vi "FTW-CSV-Variant-HeaderTraverse.vi"(0 "Variant":variant, 1 "Options":T2={"String Quotes"=FALSE, "Real Format"="%#_15g", "Timestamp Format"="%^<%Y-%m-%dT%H:%M:%S%3uZ>T", "Delimiter"=","}, 5 "Type":T1, 11 "error in":errorcluster) -> (4 "CSV String":string, 15 "error out":errorcluster)   [LabVIEW 2015]
uses:
  FTW-CSV-SerializeOptions.ctl
  <vilib>/Utility/Data Type/Type Definitions/Data Type.ctl
  <vilib>/Utility/Data Type/NI_Data Type.lvlib
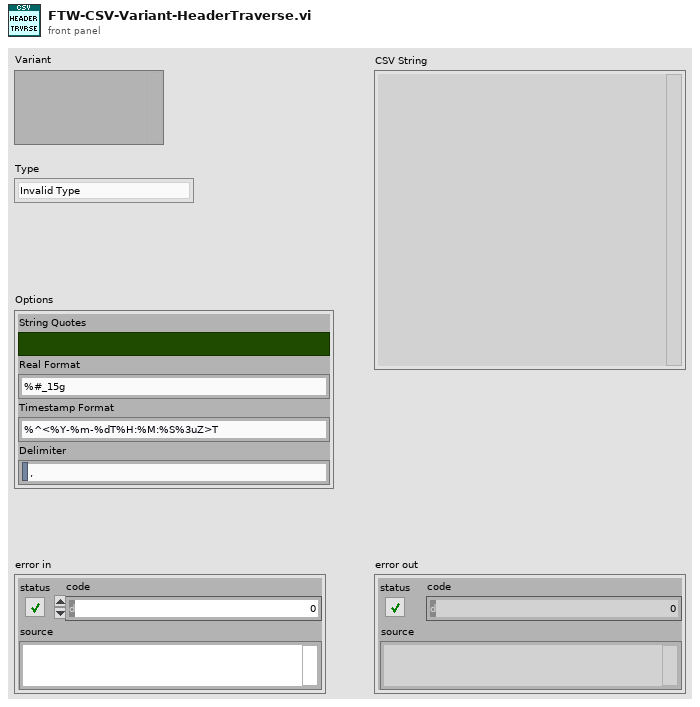
[diagram p1: front panel]
types:
  T1 = typedef "NI_Data Type.lvlib/Data Type.ctl" = enum8{"Invalid Type", "Void", "I8", "I16", "I32", "I64", "U8", "U16", "U32", "U64", "Single Float", "Double Float", "Extended Float", "Single Complex", "Double Complex", "Extended Complex", "Enum U8", "Enum U16", "Enum U32", "Enum U64", "Single Float With Unit", "Double Float With Unit", "Extended Float With Unit", "Single Complex with Unit", "Double Complex with Unit", "Extended Complex with Unit", "Boolean", "String", "Path", "Picture", "Tag", "Array", "Cluster", "Variant", "LV Variant", "Waveform", "Timestamp", "Digital Waveform", "Digital Data", "ExpressData", "Refnum", "External Data", "VI", "Poly VI", "LabVIEW Class Instance", "Fixed Point"}
  T2 = typedef "FTW-CSV-SerializeOptions.ctl" = cluster{"String Quotes":bool, "Real Format":string, "Timestamp Format":string, "Delimiter":string}
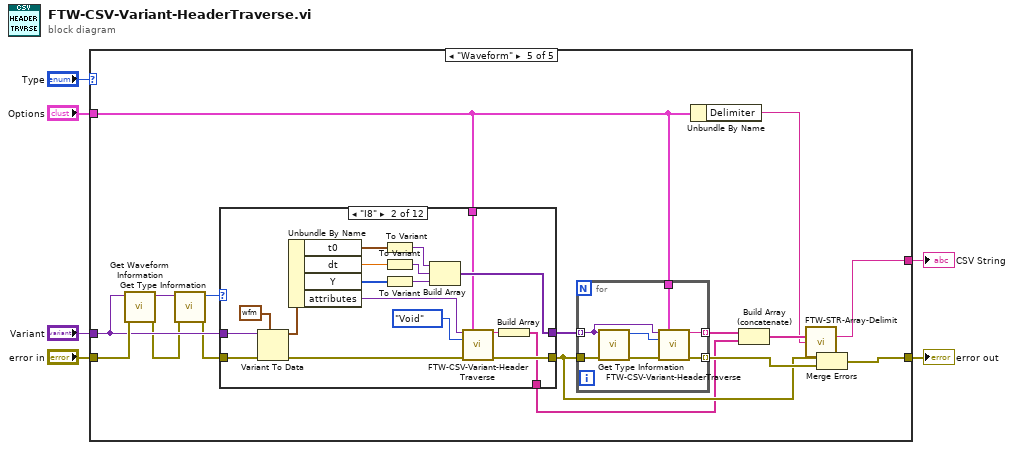
[diagram p0: block diagram]
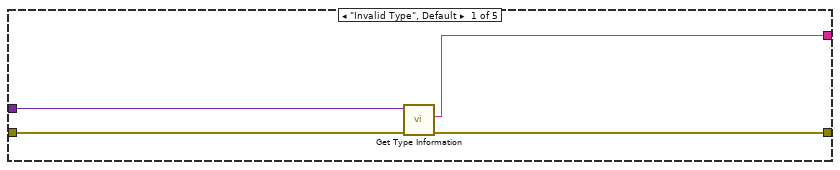
[diagram p2: hidden frame]
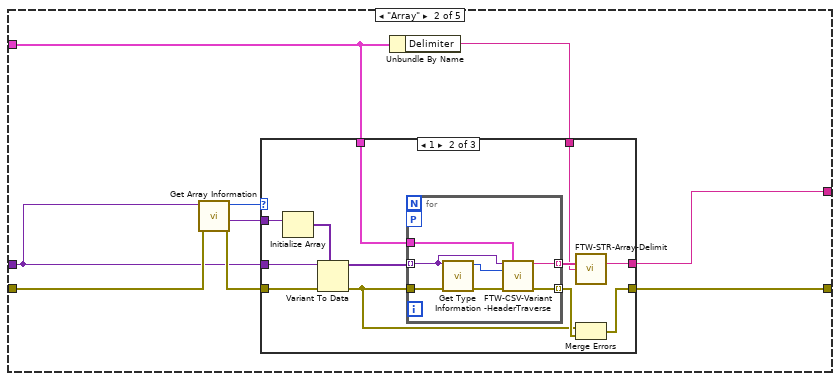
[diagram p3: hidden frame]
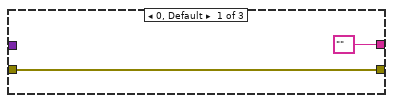
[diagram p4: hidden frame]
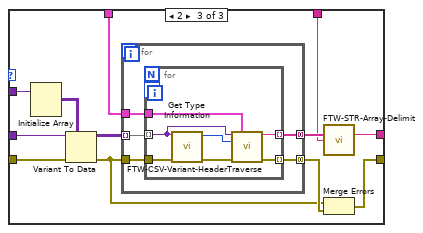
[diagram p5: hidden frame]
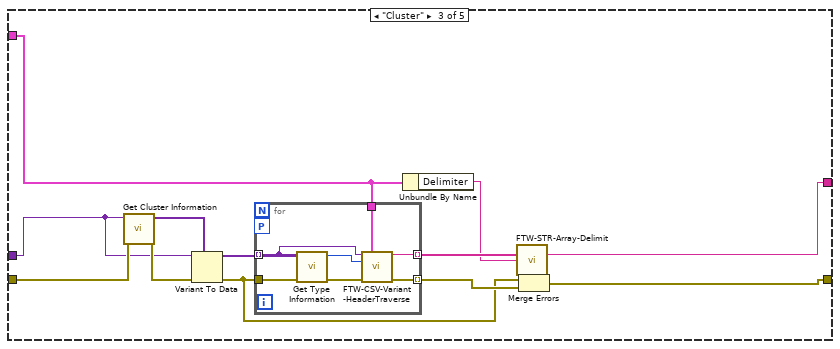
[diagram p6: hidden frame]
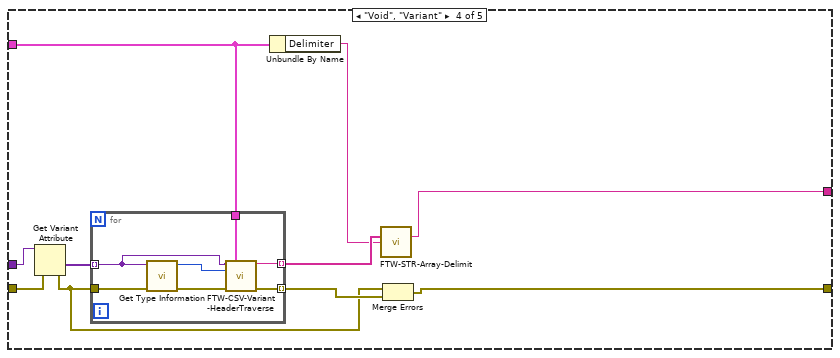
[diagram p7: hidden frame]
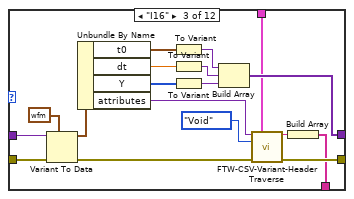
[diagram p9: hidden frame]
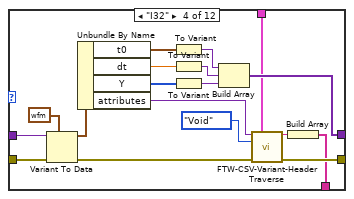
[diagram p10: hidden frame]
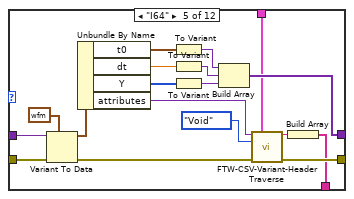
[diagram p11: hidden frame]
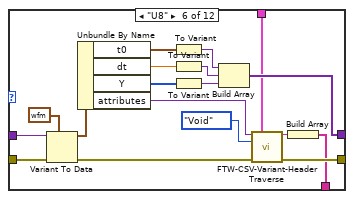
[diagram p12: hidden frame]
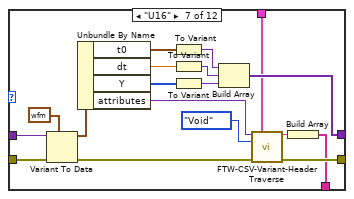
[diagram p13: hidden frame]
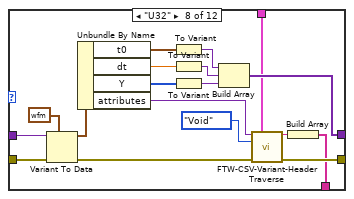
[diagram p14: hidden frame]
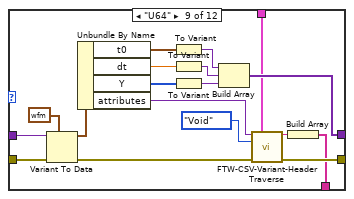
[diagram p15: hidden frame]
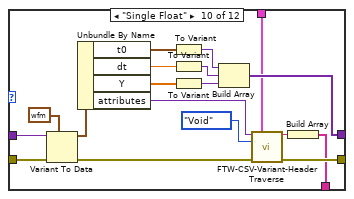
[diagram p16: hidden frame]
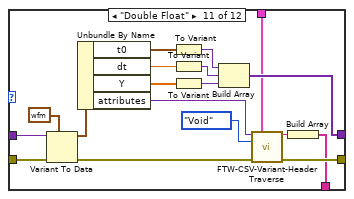
[diagram p17: hidden frame]
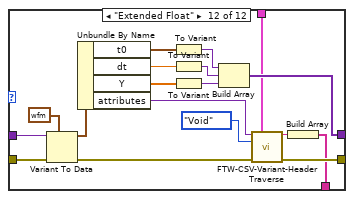
[diagram p18: hidden frame]
diagram:
  n1 = case shown="\"Waveform\"" "Type" {
    tunnel: "error in" -> [w10 w15 w68 w93 w116]
    tunnel: [w9 w14 w65 w89 w112] -> w5
    tunnel: [w7 w13 w66 w90 w113] -> w4
    tunnel: "Variant" -> [w8 w12 w67 w88 w110]
    tunnel: "Options" -> [_ w11 w69 w85 w102]
    frame "Invalid Type", Default {
      n2 = call <vilib>:"Get Type Information.vi"("error in (no error)"=w10, "Variant"=w8) -> ("error out"=w9:errorcluster, "Name"=w7:string)  [unwired: 5 in, 3 out]
    }
    frame "Array" {
      n3 = call <vilib>:"Get Array Information.vi"("error in (no error)"=w15, "Variant"=w12) -> ("error out"=w19:errorcluster, "Array Element Data Type"=w17:variant, "Number of Dimensions"=w18:i32)  [unwired: 6 in, 1 out]
      n4 = Unbundle By Name(w11) -> ("Delimiter"=w16:string)
      n5 = case shown="1" w18 {
        tunnel: [w21 w25 w44] -> w14
        tunnel: w19 -> [w21 w32 w51]
        tunnel: w17 -> [_ w28 w47]
        tunnel: ["" ("empty string") w30 w49] -> w13
        tunnel: w12 -> [_ w29 w48]
        tunnel: w11 -> [_ w23 w42]
        tunnel: w16 -> [_ w22 w41]
        frame 0, Default {
        }
        frame 1 {
          n6 = Initialize Array(w28) -> (w27:variant[])  [unwired: 1 in]
          n7 = Variant To Data(error in=w32, type=w27, Variant=w29) -> (data=w26:variant[], error out=w24:errorcluster)
          n8 = for {
            tunnel: w26 -> [w35] mode=indexing
            tunnel: [w39] -> w31 mode=indexing
            tunnel: w24 -> [w38]
            tunnel: [w40] -> w33 mode=indexing
            tunnel: w23 -> [w37]
            workers-P: _ -> [_]
            n9 = call <vilib>:"Get Type Information.vi"("error in (no error)"=w38, "Variant"=w35) -> ("error out"=w36:errorcluster, "Type"=w34:T1)  [unwired: 5 in, 3 out]
            n10 = call "FTW-CSV-Variant-HeaderTraverse.vi"("Variant"=w35, "Options"=w37, "Type"=w34, "error in"=w36) -> ("CSV String"=w39:string, "error out"=w40:errorcluster)  [unwired: 10 in]
          }
          n11 = call "FTW-STR-Array-Delimit.vi"("Array of Strings"=w31, "Delimiter"=w22) -> ("Delimited String"=w30:string)  [unwired: 13 in]
          n12 = Merge Errors(w24, w33) -> (w25:errorcluster)
        }
        frame 2 {
          n13 = Initialize Array(w47) -> (w46:variant[][])  [unwired: 2 in]
          n14 = Variant To Data(error in=w51, type=w46, Variant=w48) -> (data=w45:variant[][], error out=w43:errorcluster)
          n15 = for {
            tunnel: [w57] -> w52 mode=concatenating
            tunnel: [w56] -> w50 mode=concatenating
            tunnel: w45 -> [w55] mode=indexing
            tunnel: w43 -> [w54]
            tunnel: w42 -> [w53]
            n16 = for {
              tunnel: w55 -> [w59] mode=indexing
              tunnel: [w63] -> w56 mode=indexing
              tunnel: w54 -> [w62]
              tunnel: [w64] -> w57 mode=indexing
              tunnel: w53 -> [w61]
              workers-P: _ -> [_]
              n17 = call <vilib>:"Get Type Information.vi"("error in (no error)"=w62, "Variant"=w59) -> ("error out"=w60:errorcluster, "Type"=w58:T1)  [unwired: 5 in, 3 out]
              n18 = call "FTW-CSV-Variant-HeaderTraverse.vi"("Variant"=w59, "Options"=w61, "Type"=w58, "error in"=w60) -> ("CSV String"=w63:string, "error out"=w64:errorcluster)  [unwired: 10 in]
            }
          }
          n19 = call "FTW-STR-Array-Delimit.vi"("Array of Strings"=w50, "Delimiter"=w41) -> ("Delimited String"=w49:string)  [unwired: 13 in]
          n20 = Merge Errors(w43, w52) -> (w44:errorcluster)
        }
      }
    }
    frame "Cluster" {
      n21 = call <vilib>:"Get Cluster Information.vi"("error in (no error)"=w68, "Variant"=w67) -> ("error out"=w74:errorcluster, "Cluster Elements"=w72:variant[])  [unwired: 8 in]
      n22 = Variant To Data(error in=w74, type=w72, Variant=w67) -> (data=w71:variant[], error out=w73:errorcluster)
      n23 = for {
        tunnel: w71 -> [w78] mode=indexing
        tunnel: [w81] -> w75 mode=indexing
        tunnel: w73 -> [w83]
        tunnel: [w82] -> w76 mode=indexing
        tunnel: w69 -> [w80]
        workers-P: _ -> [_]
        n24 = call <vilib>:"Get Type Information.vi"("error in (no error)"=w83, "Variant"=w78) -> ("error out"=w79:errorcluster, "Type"=w77:T1)  [unwired: 5 in, 3 out]
        n25 = call "FTW-CSV-Variant-HeaderTraverse.vi"("Variant"=w78, "Options"=w80, "Type"=w77, "error in"=w79) -> ("CSV String"=w81:string, "error out"=w82:errorcluster)  [unwired: 10 in]
      }
      n26 = Unbundle By Name(w69) -> ("Delimiter"=w70:string)
      n27 = call "FTW-STR-Array-Delimit.vi"("Array of Strings"=w75, "Delimiter"=w70) -> ("Delimited String"=w66:string)  [unwired: 13 in]
      n28 = Merge Errors(w73, w76) -> (w65:errorcluster)
    }
    frame "Void", "Variant" {
      n29 = Get Variant Attribute(Variant=w88, error in=w93) -> (values=w86:variant[], error out=w87:errorcluster)  [unwired: 2 in, 2 out]
      n30 = for {
        tunnel: w86 -> [w95] mode=indexing
        tunnel: [w99] -> w91 mode=indexing
        tunnel: w87 -> [w97]
        tunnel: [w100] -> w92 mode=indexing
        tunnel: w85 -> [w98]
        n31 = call <vilib>:"Get Type Information.vi"("error in (no error)"=w97, "Variant"=w95) -> ("error out"=w96:errorcluster, "Type"=w94:T1)  [unwired: 5 in, 3 out]
        n32 = call "FTW-CSV-Variant-HeaderTraverse.vi"("Variant"=w95, "Options"=w98, "Type"=w94, "error in"=w96) -> ("CSV String"=w99:string, "error out"=w100:errorcluster)  [unwired: 10 in]
      }
      n33 = Unbundle By Name(w85) -> ("Delimiter"=w84:string)
      n34 = call "FTW-STR-Array-Delimit.vi"("Array of Strings"=w91, "Delimiter"=w84) -> ("Delimited String"=w90:string)  [unwired: 13 in]
      n35 = Merge Errors(w87, w92) -> (w89:errorcluster)
    }
    frame "Waveform" {
      n36 = call <vilib>:"Get Waveform Information.vi"("error in (no error)"=w116, "Variant"=w110) -> ("error out"=w107:errorcluster, "Y Array Type"=w108:variant)  [unwired: 8 in]
      n37 = call <vilib>:"Get Type Information.vi"("error in (no error)"=w107, "Variant"=w108) -> ("error out"=w106:errorcluster, "Type"=w105:T1)  [unwired: 5 in, 3 out]
      n38 = case shown="\"I8\"" w105 {
        tunnel: [w117 w123 w141 w159 w177 w195 w213 w231 w249 w267 w285 w303] -> w111
        tunnel: w110 -> [_ w127 w145 w163 w181 w199 w217 w235 w253 w271 w289 w307]
        tunnel: [_ w135 w153 w171 w189 w207 w225 w243 w261 w279 w297 w315] -> w109
        tunnel: w106 -> [w117 w131 w149 w167 w185 w203 w221 w239 w257 w275 w293 w311]
        tunnel: w102 -> [_ w122 w140 w158 w176 w194 w212 w230 w248 w266 w284 w302]
        tunnel: [_ w118 w136 w154 w172 w190 w208 w226 w244 w262 w280 w298] -> w103
        frame "Invalid Type", Default {
        }
        frame "I8" {
          n39 = Variant To Data(error in=w131, type=waveform(i8) {"t0"=timestamp(0 s since 1904-01-01), "dt"=1.0, "Y"=[]} ("Waveform"), Variant=w127) -> (data=w125:waveform(i8), error out=w124:errorcluster)
          n40 = Unbundle By Name(w125) -> ("t0"=w130:timestamp, "dt"=w129:dbl, "Y"=w128:i8[], "attributes"=w121:variant)
          n41 = To Variant(anything=w130) -> (Variant=w134:variant)
          n42 = To Variant(anything=w129) -> (Variant=w133:variant)
          n43 = To Variant(anything=w128) -> (Variant=w132:variant)
          n44 = Build Array(w134, w133, w132) -> (w135:variant[])
          n45 = call "FTW-CSV-Variant-HeaderTraverse.vi"("Variant"=w121, "Options"=w122, "Type"=Data_Type."Void", "error in"=w124) -> ("CSV String"=w119:string, "error out"=w123:errorcluster)  [unwired: 10 in]
          n46 = Build Array(w119) -> (w118:string[])
        }
        frame "I16" {
          n47 = Variant To Data(error in=w149, type=waveform(i16) {"t0"=timestamp(0 s since 1904-01-01), "dt"=1.0, "Y"=[]} ("Waveform"), Variant=w145) -> (data=w143:waveform(i16), error out=w142:errorcluster)
          n48 = Unbundle By Name(w143) -> ("t0"=w148:timestamp, "dt"=w147:dbl, "Y"=w146:i16[], "attributes"=w139:variant)
          n49 = To Variant(anything=w148) -> (Variant=w152:variant)
          n50 = To Variant(anything=w147) -> (Variant=w151:variant)
          n51 = To Variant(anything=w146) -> (Variant=w150:variant)
          n52 = Build Array(w152, w151, w150) -> (w153:variant[])
          n53 = call "FTW-CSV-Variant-HeaderTraverse.vi"("Variant"=w139, "Options"=w140, "Type"=Data_Type."Void", "error in"=w142) -> ("CSV String"=w137:string, "error out"=w141:errorcluster)  [unwired: 10 in]
          n54 = Build Array(w137) -> (w136:string[])
        }
        frame "I32" {
          n55 = Variant To Data(error in=w167, type=waveform(i32) {"t0"=timestamp(0 s since 1904-01-01), "dt"=1.0, "Y"=[]} ("Waveform"), Variant=w163) -> (data=w161:waveform(i32), error out=w160:errorcluster)
          n56 = Unbundle By Name(w161) -> ("t0"=w166:timestamp, "dt"=w165:dbl, "Y"=w164:i32[], "attributes"=w157:variant)
          n57 = To Variant(anything=w166) -> (Variant=w170:variant)
          n58 = To Variant(anything=w165) -> (Variant=w169:variant)
          n59 = To Variant(anything=w164) -> (Variant=w168:variant)
          n60 = Build Array(w170, w169, w168) -> (w171:variant[])
          n61 = call "FTW-CSV-Variant-HeaderTraverse.vi"("Variant"=w157, "Options"=w158, "Type"=Data_Type."Void", "error in"=w160) -> ("CSV String"=w155:string, "error out"=w159:errorcluster)  [unwired: 10 in]
          n62 = Build Array(w155) -> (w154:string[])
        }
        frame "I64" {
          n63 = Variant To Data(error in=w185, type=waveform(i64) {"t0"=timestamp(0 s since 1904-01-01), "dt"=1.0, "Y"=[]} ("Waveform"), Variant=w181) -> (data=w179:waveform(i64), error out=w178:errorcluster)
          n64 = Unbundle By Name(w179) -> ("t0"=w184:timestamp, "dt"=w183:dbl, "Y"=w182:i64[], "attributes"=w175:variant)
          n65 = To Variant(anything=w184) -> (Variant=w188:variant)
          n66 = To Variant(anything=w183) -> (Variant=w187:variant)
          n67 = To Variant(anything=w182) -> (Variant=w186:variant)
          n68 = Build Array(w188, w187, w186) -> (w189:variant[])
          n69 = call "FTW-CSV-Variant-HeaderTraverse.vi"("Variant"=w175, "Options"=w176, "Type"=Data_Type."Void", "error in"=w178) -> ("CSV String"=w173:string, "error out"=w177:errorcluster)  [unwired: 10 in]
          n70 = Build Array(w173) -> (w172:string[])
        }
        frame "U8" {
          n71 = Variant To Data(error in=w203, type=waveform(u8) {"t0"=timestamp(0 s since 1904-01-01), "dt"=1.0, "Y"=[]} ("Waveform"), Variant=w199) -> (data=w197:waveform(u8), error out=w196:errorcluster)
          n72 = Unbundle By Name(w197) -> ("t0"=w202:timestamp, "dt"=w201:dbl, "Y"=w200:u8[], "attributes"=w193:variant)
          n73 = To Variant(anything=w202) -> (Variant=w206:variant)
          n74 = To Variant(anything=w201) -> (Variant=w205:variant)
          n75 = To Variant(anything=w200) -> (Variant=w204:variant)
          n76 = Build Array(w206, w205, w204) -> (w207:variant[])
          n77 = call "FTW-CSV-Variant-HeaderTraverse.vi"("Variant"=w193, "Options"=w194, "Type"=Data_Type."Void", "error in"=w196) -> ("CSV String"=w191:string, "error out"=w195:errorcluster)  [unwired: 10 in]
          n78 = Build Array(w191) -> (w190:string[])
        }
        frame "U16" {
          n79 = Variant To Data(error in=w221, type=waveform(u16) {"t0"=timestamp(0 s since 1904-01-01), "dt"=1.0, "Y"=[]} ("Waveform"), Variant=w217) -> (data=w215:waveform(u16), error out=w214:errorcluster)
          n80 = Unbundle By Name(w215) -> ("t0"=w220:timestamp, "dt"=w219:dbl, "Y"=w218:u16[], "attributes"=w211:variant)
          n81 = To Variant(anything=w220) -> (Variant=w224:variant)
          n82 = To Variant(anything=w219) -> (Variant=w223:variant)
          n83 = To Variant(anything=w218) -> (Variant=w222:variant)
          n84 = Build Array(w224, w223, w222) -> (w225:variant[])
          n85 = call "FTW-CSV-Variant-HeaderTraverse.vi"("Variant"=w211, "Options"=w212, "Type"=Data_Type."Void", "error in"=w214) -> ("CSV String"=w209:string, "error out"=w213:errorcluster)  [unwired: 10 in]
          n86 = Build Array(w209) -> (w208:string[])
        }
        frame "U32" {
          n87 = Variant To Data(error in=w239, type=waveform(u32) {"t0"=timestamp(0 s since 1904-01-01), "dt"=1.0, "Y"=[]} ("Waveform"), Variant=w235) -> (data=w233:waveform(u32), error out=w232:errorcluster)
          n88 = Unbundle By Name(w233) -> ("t0"=w238:timestamp, "dt"=w237:dbl, "Y"=w236:u32[], "attributes"=w229:variant)
          n89 = To Variant(anything=w238) -> (Variant=w242:variant)
          n90 = To Variant(anything=w237) -> (Variant=w241:variant)
          n91 = To Variant(anything=w236) -> (Variant=w240:variant)
          n92 = Build Array(w242, w241, w240) -> (w243:variant[])
          n93 = call "FTW-CSV-Variant-HeaderTraverse.vi"("Variant"=w229, "Options"=w230, "Type"=Data_Type."Void", "error in"=w232) -> ("CSV String"=w227:string, "error out"=w231:errorcluster)  [unwired: 10 in]
          n94 = Build Array(w227) -> (w226:string[])
        }
        frame "U64" {
          n95 = Variant To Data(error in=w257, type=waveform(u64) {"t0"=timestamp(0 s since 1904-01-01), "dt"=1.0, "Y"=[]} ("Waveform"), Variant=w253) -> (data=w251:waveform(u64), error out=w250:errorcluster)
          n96 = Unbundle By Name(w251) -> ("t0"=w256:timestamp, "dt"=w255:dbl, "Y"=w254:u64[], "attributes"=w247:variant)
          n97 = To Variant(anything=w256) -> (Variant=w260:variant)
          n98 = To Variant(anything=w255) -> (Variant=w259:variant)
          n99 = To Variant(anything=w254) -> (Variant=w258:variant)
          n100 = Build Array(w260, w259, w258) -> (w261:variant[])
          n101 = call "FTW-CSV-Variant-HeaderTraverse.vi"("Variant"=w247, "Options"=w248, "Type"=Data_Type."Void", "error in"=w250) -> ("CSV String"=w245:string, "error out"=w249:errorcluster)  [unwired: 10 in]
          n102 = Build Array(w245) -> (w244:string[])
        }
        frame "Single Float" {
          n103 = Variant To Data(error in=w275, type=waveform(sgl) {"t0"=timestamp(0 s since 1904-01-01), "dt"=1.0, "Y"=[]} ("Waveform"), Variant=w271) -> (data=w269:waveform(sgl), error out=w268:errorcluster)
          n104 = Unbundle By Name(w269) -> ("t0"=w274:timestamp, "dt"=w273:dbl, "Y"=w272:sgl[], "attributes"=w265:variant)
          n105 = To Variant(anything=w274) -> (Variant=w278:variant)
          n106 = To Variant(anything=w273) -> (Variant=w277:variant)
          n107 = To Variant(anything=w272) -> (Variant=w276:variant)
          n108 = Build Array(w278, w277, w276) -> (w279:variant[])
          n109 = call "FTW-CSV-Variant-HeaderTraverse.vi"("Variant"=w265, "Options"=w266, "Type"=Data_Type."Void", "error in"=w268) -> ("CSV String"=w263:string, "error out"=w267:errorcluster)  [unwired: 10 in]
          n110 = Build Array(w263) -> (w262:string[])
        }
        frame "Double Float" {
          n111 = Variant To Data(error in=w293, type=waveform(dbl) {"t0"=timestamp(0 s since 1904-01-01), "dt"=1.0, "Y"=[]} ("Waveform"), Variant=w289) -> (data=w287:waveform(dbl), error out=w286:errorcluster)
          n112 = Unbundle By Name(w287) -> ("t0"=w292:timestamp, "dt"=w291:dbl, "Y"=w290:dbl[], "attributes"=w283:variant)
          n113 = To Variant(anything=w292) -> (Variant=w296:variant)
          n114 = To Variant(anything=w291) -> (Variant=w295:variant)
          n115 = To Variant(anything=w290) -> (Variant=w294:variant)
          n116 = Build Array(w296, w295, w294) -> (w297:variant[])
          n117 = call "FTW-CSV-Variant-HeaderTraverse.vi"("Variant"=w283, "Options"=w284, "Type"=Data_Type."Void", "error in"=w286) -> ("CSV String"=w281:string, "error out"=w285:errorcluster)  [unwired: 10 in]
          n118 = Build Array(w281) -> (w280:string[])
        }
        frame "Extended Float" {
          n119 = Variant To Data(error in=w311, type=waveform(ext) {"t0"=timestamp(0 s since 1904-01-01), "dt"=1.0, "Y"=[]} ("Waveform"), Variant=w307) -> (data=w305:waveform(ext), error out=w304:errorcluster)
          n120 = Unbundle By Name(w305) -> ("t0"=w310:timestamp, "dt"=w309:dbl, "Y"=w308:ext[], "attributes"=w301:variant)
          n121 = To Variant(anything=w310) -> (Variant=w314:variant)
          n122 = To Variant(anything=w309) -> (Variant=w313:variant)
          n123 = To Variant(anything=w308) -> (Variant=w312:variant)
          n124 = Build Array(w314, w313, w312) -> (w315:variant[])
          n125 = call "FTW-CSV-Variant-HeaderTraverse.vi"("Variant"=w301, "Options"=w302, "Type"=Data_Type."Void", "error in"=w304) -> ("CSV String"=w299:string, "error out"=w303:errorcluster)  [unwired: 10 in]
          n126 = Build Array(w299) -> (w298:string[])
        }
      }
      n127 = for {
        tunnel: w109 -> [w317] mode=indexing
        tunnel: [w320] -> w114 mode=indexing
        tunnel: w111 -> [w322]
        tunnel: [w321] -> w115 mode=indexing
        tunnel: w102 -> [w319]
        n128 = call <vilib>:"Get Type Information.vi"("error in (no error)"=w322, "Variant"=w317) -> ("error out"=w318:errorcluster, "Type"=w316:T1)  [unwired: 5 in, 3 out]
        n129 = call "FTW-CSV-Variant-HeaderTraverse.vi"("Variant"=w317, "Options"=w319, "Type"=w316, "error in"=w318) -> ("CSV String"=w320:string, "error out"=w321:errorcluster)  [unwired: 10 in]
      }
      n130 = Unbundle By Name(w102) -> ("Delimiter"=w101:string)
      n131 = Build Array (concatenate)(w114, w103) -> (w104:string[])
      n132 = call "FTW-STR-Array-Delimit.vi"("Array of Strings"=w104, "Delimiter"=w101) -> ("Delimited String"=w113:string)  [unwired: 13 in]
      n133 = Merge Errors(w111, w115) -> (w112:errorcluster)
    }
  }
  "error out" <- w5
  "CSV String" <- w4
